vi "Read Module Slot.vi"(8 "error in":errorcluster, 9 "slot":i32, 10 "chuck":i32, 11 "WorkTable in":refnum<class "WorkTable Class.lvclass">) -> (0 "error out":errorcluster, 2 "Module Slot":T1, 3 "WorkTable out":refnum<class "WorkTable Class.lvclass">)   [LabVIEW 2011, in "WorkTable Class.lvclass"]
uses:
  WorkTable Class.lvclass
  Type Definitions/Worktable_Module Slot.ctl
  Vec3d Class/Vec3d Class.lvclass
  Orient3d Class/Orient3d Class.lvclass
  Utils/Type Definitions/Position_Orientation.ctl
  WorkTable Class.lvclass/WorkTable Class.ctl
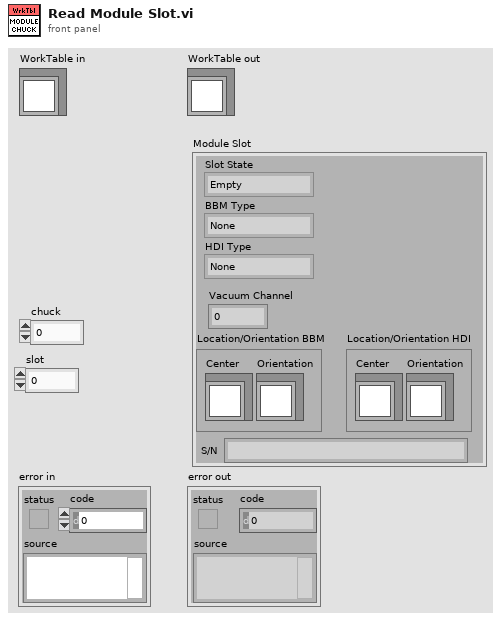
[diagram p1: front panel]
types:
  T1 = typedef "Worktable_Module Slot.ctl" = cluster{"Slot State":enum16{"Empty", "Unglued", "Stamped", "PartOnTop", "Weighted", "Unpotted", "Potted"}, "BBM Type":enum16{"None", "BBM", "GlassSlide"}, "HDI Type":enum16{"None", "HDI", "Polyimide"}, "Vacuum Channel":u8, "Location/Orientation BBM":T2, "Location/Orientation HDI":T2, "S/N":string}
  T2 = typedef "Position_Orientation.ctl" = cluster{"Center":refnum<class "Vec3d Class.lvclass">, "Orientation":refnum<class "Orient3d Class.lvclass">}
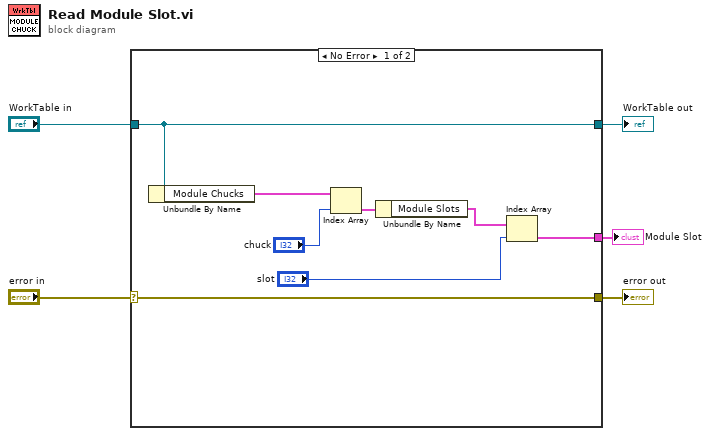
[diagram p0: block diagram]
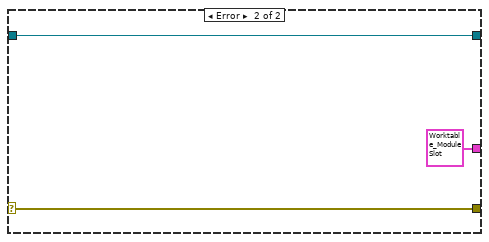
[diagram p2: hidden frame]
diagram:
  n1 = case shown="No Error" "error in" {
    selector: "error in" -> [w13 w15]
    tunnel: [w13 w15] -> w4
    tunnel: [w12 w16] -> w2
    tunnel: "WorkTable in" -> [w12 w16]
    tunnel: [w6 T1 {"Slot State"=enum."Empty", "BBM Type"=enum."None", "HDI Type"=enum."None", "Vacuum Channel"=0, "Location/Orientation BBM"={"Center"=refnum, "Orientation"=refnum}, "Location/Orientation HDI"={"Center"=refnum, "Orientation"=refnum}, "S/N"=""} ("BBM Slot")] -> w1
    frame No Error {
      n2 = Unbundle By Name(w12) -> ("Module Chucks"=w11:cluster{"Module Slots":T1[]}[])
      n3 = Index Array(array=w11, index="chuck") -> (element=w9:cluster{"Module Slots":T1[]})
      n4 = Unbundle By Name(w9) -> ("Module Slots"=w8:T1[])
      n5 = Index Array(array=w8, index="slot") -> (element=w6:T1)
    }
    frame Error {
    }
  }
  "error out" <- w4
  "WorkTable out" <- w2
  "Module Slot" <- w1
